vi "XY Graph Order Plot Axis.vi"(8 "Order (ascending)":enum16{"ascending", "descending"}(ring), 10 "Plot Values":dbl[](array[numeric]), 11 "Plot Axis":dbl[](array[numeric])) -> (2 "Ordered Axis Plot Values":dbl[](array[numeric]), 3 "Ordered Plot Axis":dbl[](array[numeric]))   [LabVIEW 2021, in "XY Graph Add-Ons.lvlib"]
uses:
  XY Graph Add-Ons.lvlib
  <userlib>/_OpenG.lib/array/array.llb/Sort 1D Array (DBL)__ogtk.vi
  <userlib>/_OpenG.lib/array/array.llb/Reorder 1D Array2 (DBL)__ogtk.vi
  <userlib>/_OpenG.lib/array/array.llb/openg_array.lvlib
panel:
  # "see the AlliGator License on the block diagram (Ctrl+E or Window:Show Block Diagram)"
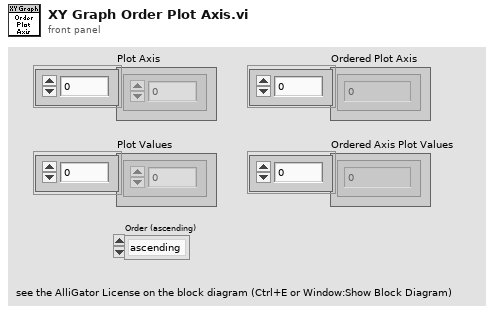
[diagram p1: front panel]
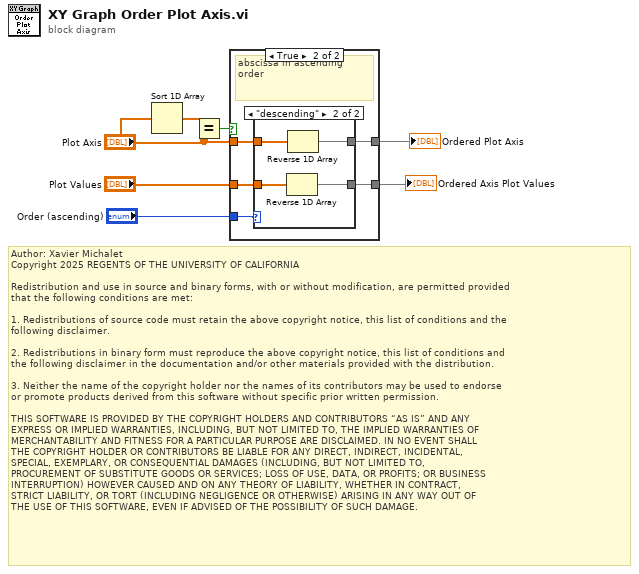
[diagram p0: block diagram]
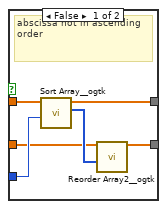
[diagram p2: hidden frame]
diagram:
  # "Author: Xavier Michalet\nCopyright 2025 REGENTS OF THE UNIVERSITY OF CALIFORNIA\n\nRedistribution and use in source and binary forms, with or without modification, are permitted provided\nthat the following conditions are met:\n\n1. Redistributions of source code must retain the above copyright notice, this list of conditions and the\nfollowing disclaimer.\n\n2. Redistributions in binary form must reproduce the above copyright notice, this list of conditions and\nthe following disclaimer in the documentation and/or other materials provided with the distribution.\n\n3. Neither the name of the copyright holder nor the names of its contributors may be used to endorse \nor promote products derived from this software without specific prior written permission.\n\nTHIS SOFTWARE IS PROVIDED BY THE COPYRIGHT HOLDERS AND CONTRIBUTORS “AS IS” AND ANY \nEXPRESS OR IMPLIED WARRANTIES, INCLUDING, BUT NOT LIMITED TO, THE IMPLIED WARRANTIES OF\nMERCHANTABILITY AND FITNESS FOR A PARTICULAR PURPOSE ARE DISCLAIMED. IN NO EVENT SHALL\nTHE COPYRIGHT HOLDER OR CONTRIBUTORS BE LIABLE FOR ANY DIRECT, INDIRECT, INCIDENTAL, \nSPECIAL, EXEMPLARY, OR CONSEQUENTIAL DAMAGES (INCLUDING, BUT NOT LIMITED TO, \nPROCUREMENT OF SUBSTITUTE GOODS OR SERVICES; LOSS OF USE, DATA, OR PROFITS; OR BUSINESS\nINTERRUPTION) HOWEVER CAUSED AND ON ANY THEORY OF LIABILITY, WHETHER IN CONTRACT, \nSTRICT LIABILITY, OR TORT (INCLUDING NEGLIGENCE OR OTHERWISE) ARISING IN ANY WAY OUT OF\nTHE USE OF THIS SOFTWARE, EVEN IF ADVISED OF THE POSSIBILITY OF SUCH DAMAGE."
  n1 = Sort 1D Array(array="Plot Axis") -> (sorted array=w7:dbl[])
  n2 = Equal?(x=w7, y="Plot Axis") -> (x = y?=w6:bool)
  n3 = case shown="True" w6 {
    tunnel: "Plot Values" -> [w9 w16]
    tunnel: [w11 w15] -> w3
    tunnel: "Plot Axis" -> [w13 w17]
    tunnel: [w8 w14] -> w2
    tunnel: "Order (ascending)" -> [w12 w18]
    frame False {
      # "abscissa not in ascending order"
      n4 = call-poly <userlib>:"Sort Array__ogtk.vi"("Order"=w12, "Array in"=w13) -> ("Sorted Pointers"=w10:i32[], "Sorted Array out"=w11:dbl[])  [unwired: 8 in]
      n5 = call-poly <userlib>:"Reorder Array2__ogtk.vi"("indices"=w10, "array"=w9) -> ("reordered array"=w8:dbl[])  [unwired: 9 in]
    }
    frame True {
      # "abscissa in ascending order"
      n6 = case shown="\"descending\"" w18 {
        tunnel: w17 -> [w20 w24]
        tunnel: w16 -> [w19 w22]
        tunnel: [w20 w23] -> w15
        tunnel: [w19 w21] -> w14
        frame "ascending", Default {
        }
        frame "descending" {
          n7 = Reverse 1D Array(array=w22) -> (reversed array=w21:dbl[])
          n8 = Reverse 1D Array(array=w24) -> (reversed array=w23:dbl[])
        }
      }
    }
  }
  "Ordered Plot Axis" <- w3
  "Ordered Axis Plot Values" <- w2
